vi "Read WiFi Config.vi"() -> (0 "error out":errorcluster={"status"=TRUE, "code"=7227, "source"="LJM_OpenS.vi"})   [LabVIEW 2017]
panel:
  in  "Case Constant\n(See Context Help)":bool
  out "Default SSID":string
  out "Default SSID":string
  out "Current SSID":string
  out "Values (other)":dbl[](array[numeric]) format="%.2f"
  in  "Names (other)":string[](array[string])=["WIFI_STATUS", "WIFI_RSSI", "WIFI_DHCP_ENABLE_DEFAULT"]
  out "NumberToIP":string[](array[string])
  out "Error String":string="LabJack Error #1227:  LJME_DEVICE_NOT_FOUND occured at LJM_OpenS.vi"
  out "ConnectionType Out":i32
  out "DeviceType Out":i32
  in  "Identifier":string="192.168.0.101"
  in  "ConnectionType":string="WIFI"
  in  "DeviceType":string="T7"
  out "Values (IP)":dbl[](array[numeric]) format="%.2f"
  in  "Names (IP)":string[](array[string])=["WIFI_IP", "WIFI_SUBNET", "WIFI_GATEWAY", "WIFI_IP_DEFAULT", "WIFI_SUBNET_DEFAULT", "WIFI_GATEWAY_DEFAULT"]
  # "// WiFi Status Codes:\n#define WIFI_ASSOCIATED                          2900\n#define WIFI_ASSOCIATING                        2901\n#define WIFI_ASSOCIATION_FAILED         2902\n#define WIFI_UNPOWERED                         2903\n#define WIFI_BOOTING_UP                         2904\n#define WIFI_COULD_NOT_START             2905\n#define WIFI_APPLYING_SETTINGS            2906\n#define WIFI_DHCP_STARTED                     2907\n#define WIFI_OTHER                                     2909"
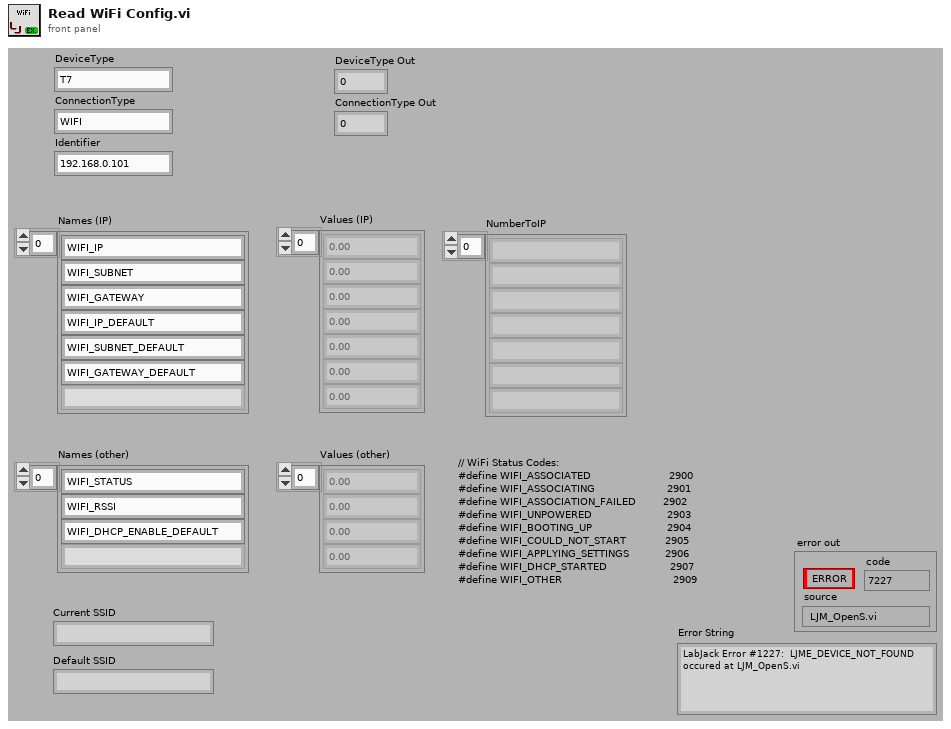
[diagram p1: front panel]
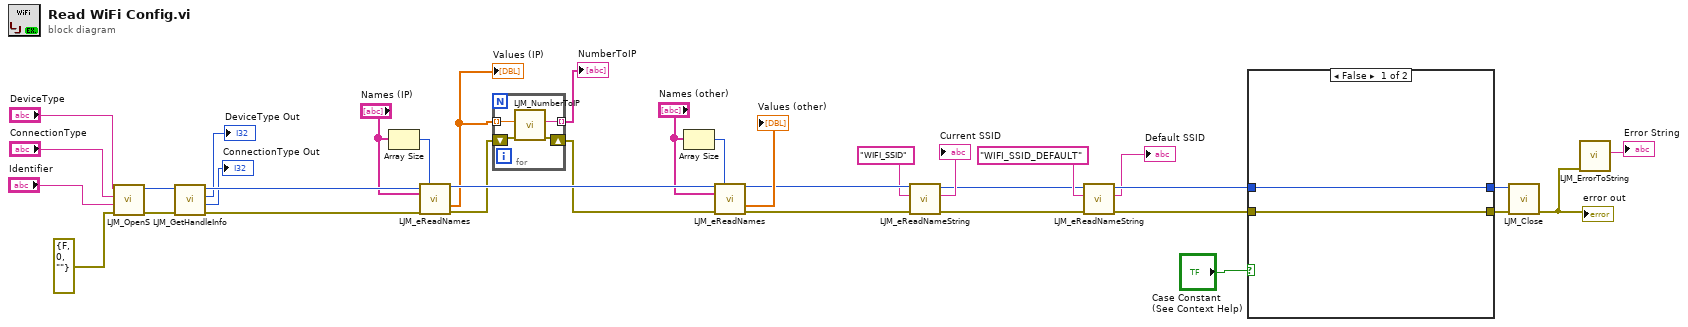
[diagram p0: block diagram]
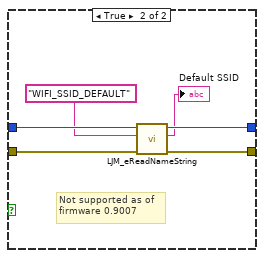
[diagram p2: hidden frame]
diagram:
  n1 = call <userlib>:"LJM_OpenS.vi"("error in"=errorcluster {"status"=FALSE, "code"=0, "source"=""} ("error in (no error)"), "Identifier"="Identifier", "ConnectionType"="ConnectionType", "DeviceType"="DeviceType") -> ("error out"=w34:errorcluster, "Handle"=w32:i32)  [unwired: 6 in]
  n2 = call <userlib>:"LJM_GetHandleInfo.vi"("error in"=w34, "Handle In"=w32) -> ("error out"=w33:errorcluster, "ConnectionType"=→"ConnectionType Out":i32, "DeviceType"=→"DeviceType Out":i32, "Handle Out"=w31:i32)  [unwired: 2 in, 4 out]
  n3 = Array Size(array="Names (IP)") -> (size(s)=w22:i32)
  n4 = call "LJM_eReadNames.vi"("Handle In"=w31, "NumFrames"=w22, "aNames"="Names (IP)", "error in"=w33) -> ("Handle Out"=w20:i32, "aValuesOut"=w11:dbl[], "error out"=w9:errorcluster)  [unwired: 8 in, 1 out]
  "Values (IP)" <- w11
  n5 = for {
    tunnel: w11 -> [w39] mode=indexing
    tunnel: [w38] -> w10 mode=indexing
    shift-right: [w36] -> w8
    shift-left: w9 -> [w37]
    n6 = call "LJM_NumberToIP.vi"("error in"=w37, "Number"=w39) -> ("error out"=w36:errorcluster, "IPv4String"=w38:string)  [unwired: 8 in]
  }
  "NumberToIP" <- w10
  n7 = Array Size(array="Names (other)") -> (size(s)=w21:i32)
  n8 = call "LJM_eReadNames.vi"("Handle In"=w20, "NumFrames"=w21, "aNames"="Names (other)", "error in"=w8) -> ("Handle Out"=w17:i32, "aValuesOut"=→"Values (other)":dbl[], "error out"=w16:errorcluster)  [unwired: 8 in, 1 out]
  n9 = call "LJM_eReadNameString.vi"("error in"=w16, "Name"="WIFI_SSID", "Handle In"=w17) -> ("error out"=w4:errorcluster, "String"=→"Current SSID":string, "Handle Out"=w5:i32)  [unwired: 6 in]
  n10 = call "LJM_eReadNameString.vi"("error in"=w4, "Name"="WIFI_SSID_DEFAULT", "Handle In"=w5) -> ("error out"=w3:errorcluster, "String"=→"Default SSID":string, "Handle Out"=w2:i32)  [unwired: 6 in]
  n11 = case shown="False" "Case Constant\n(See Context Help)" {
    tunnel: w2 -> [w41 w47]
    tunnel: w3 -> [w40 w46]
    tunnel: [w40 w45] -> w13
    tunnel: [w41 w44] -> w12
    frame False {
    }
    frame True {
      # "Not supported as of\nfirmware 0.9007"
      n12 = call "LJM_eReadNameString.vi"("error in"=w46, "Name"="WIFI_SSID_DEFAULT", "Handle In"=w47) -> ("error out"=w45:errorcluster, "String"=→"Default SSID":string, "Handle Out"=w44:i32)  [unwired: 6 in]
    }
  }
  n13 = call <userlib>:"LJM_Close.vi"("error in"=w13, "Handle"=w12) -> ("error out"=w25:errorcluster)  [unwired: 9 in]
  "error out" <- w25
  n14 = call <userlib>:"LJM_ErrorToString.vi"("error in"=w25) -> ("String"=→"Error String":string)  [unwired: 10 in]
